vi "Agilent Reset IP.vi"(8 "error in (no error)":errorcluster, 11 "VISA Resource Name":refnum<visa-resource-name>="A-34972A") -> (0 "error out":errorcluster, 3 "VISA Resource Name Out":refnum<visa-resource-name>)   [LabVIEW 2009]
doc: "This VI allows you to save or recall an instrument setup state. You can save a current configuration to states 0-5, or you can recall a setup from states 0-5 or the instrument's preset state."
panel:
  in  "IPAD":string="10.2.0.32"
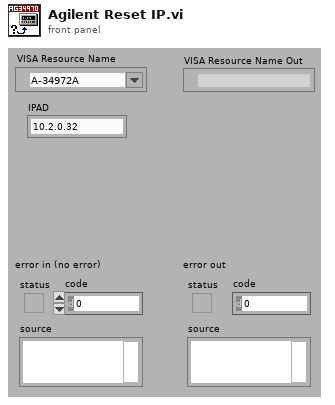
[diagram p1: front panel]
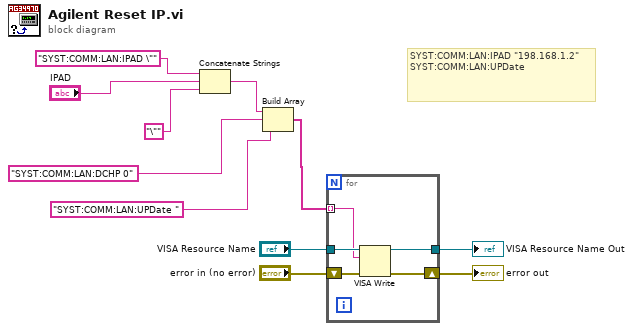
[diagram p0: block diagram]
diagram:
  # "SYST:COMM:LAN:IPAD \"198.168.1.2\" \nSYST:COMM:LAN:UPDate"
  n1 = Concatenate Strings("SYST:COMM:LAN:IPAD \"" ("write buffer"), "IPAD", "\"" ("write buffer")) -> (w4:string)
  n2 = Build Array(w4, "SYST:COMM:LAN:DCHP 0" ("write buffer"), "SYST:COMM:LAN:UPDate " ("write buffer")) -> (w3:string[])
  n3 = for {
    tunnel: "VISA Resource Name" -> [w16]
    tunnel: [w13] -> w8
    shift-right: [w14] -> w9
    shift-left: "error in (no error)" -> [w15]
    tunnel: w3 -> [w12] mode=indexing
    n4 = VISA Write(VISA resource name=w16, write buffer=w12, error in (no error)=w15) -> (VISA resource name out=w13:refnum<visa-resource-name>, error out=w14:errorcluster)  [unwired: 1 out]
  }
  "error out" <- w9
  "VISA Resource Name Out" <- w8
